vi "update_waypoints.vi"(11 "Mission in":refnum<class "Mission.lvclass">) -> (3 "Mission out":refnum<class "Mission.lvclass">)   [LabVIEW 2011, in "Mission.lvclass"]
uses:
  Mission.lvclass
  2 Globals/2 Global.vi
  Waypoint/Waypoint.lvclass
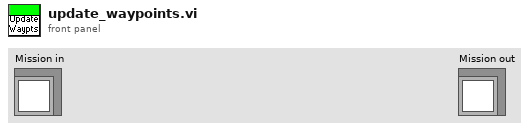
[diagram p1: front panel]
types:
  T1 = enum16{"Round Buoy", "Drive", "Pass Buoys", "Station Keeping"}
  T2 = typedef "UTM Location.ctl" = cluster{"UTM Zone":dbl, "Hemisphere":enum16{"North", "South"}, "East":dbl, "North":dbl}
  T3 = typedef "Waypoints List.ctl" = refnum<class "Waypoint.lvclass">[]
  T4 = typedef "Current Waypoint.ctl" = i32
  T5 = typedef "UTM Circle.ctl" = cluster{"UTM Zone":dbl, "Hemisphere":enum16{"North", "South"}, "East":dbl, "North":dbl, "Radius":dbl}
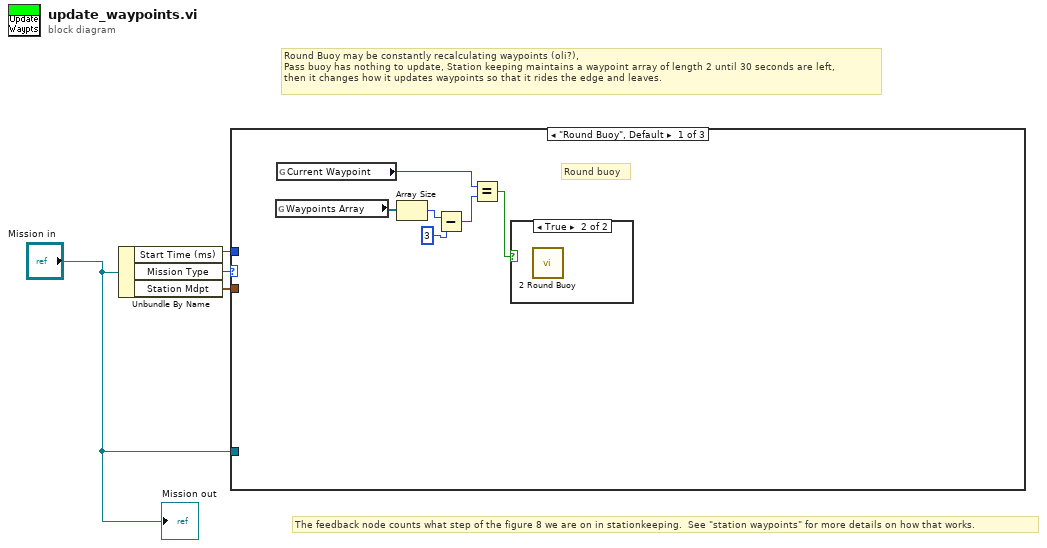
[diagram p0: block diagram]
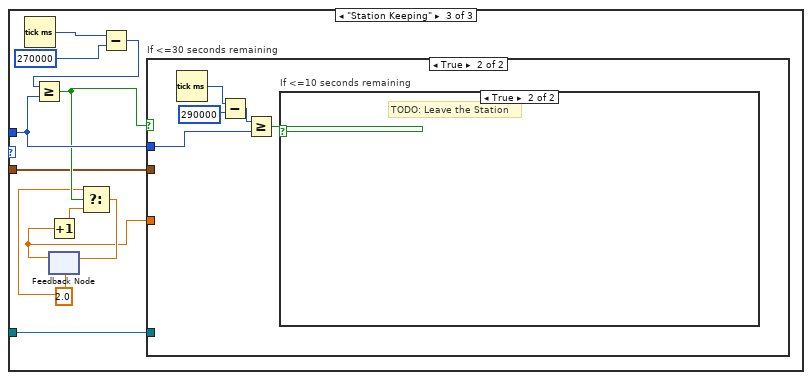
[diagram p4: hidden frame]
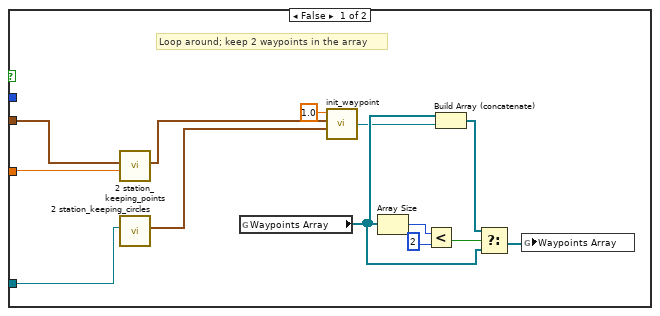
[diagram p5: hidden frame]
diagram:
  # "The feedback node counts what step of the figure 8 we are on in stationkeeping.  See \"station waypoints\" for more details on how that works."
  # "Round Buoy may be constantly recalculating waypoints (oli?),\nPass buoy has nothing to update, Station keeping maintains a waypoint array of length 2 until 30 seconds are left,\nthen it changes how it updates waypoints so that it rides the edge and leaves."
  n1 = Unbundle By Name("Mission in") -> ("Start Time (ms)"=w3:u32, "Mission Type"=w4:T1, "Station Mdpt"=w1:T2)
  n2 = case shown="\"Round Buoy\", Default" w4 {
    tunnel: w3 -> [_ _ w19]
    tunnel: "Mission in" -> [_ _ w12]
    tunnel: w1 -> [_ _ w11]
    frame "Round Buoy", Default {
      # "Round buoy"
      n3 = global read "2 Global.vi" "Waypoints Array"() -> (w9:T3)
      n4 = global read "2 Global.vi" "Current Waypoint"() -> (w7:T4)
      n5 = Array Size(array=w9) -> (size(s)=w8:i32)
      n6 = Subtract(x=w8, y=3) -> (x-y=w6:i32)
      n7 = Equal?(x=w7, y=w6) -> (x = y?=w5:bool)
      n8 = case shown="True" w5 {
        frame False {
        }
        frame True {
          n9 = call "2 Round Buoy.vi"() -> ()  [unwired: 12 in]
        }
      }
    }
    frame "Pass Buoys" {
    }
    frame "Station Keeping" {
      w15 = 2.0
      n10 = Tick Count (ms)() -> (millisecond timer value=w21:u32)
      n11 = feedback #1(w15) -> (w13:dbl)
      n12 = Increment(x=w13) -> (x+1=w16:dbl)
      n13 = Subtract(x=w21, y=u32 270000) -> (x-y=w18:u32)
      n14 = Greater Or Equal?(x=w18, y=w19) -> (x >= y?=w17:bool)
      n15 = Select(t=w15, s=w17, f=w16) -> (s? t:f=w14:dbl)
      n16 = feedback-in #1(w14) -> ()
      n17 = case "If <=30 seconds remaining" shown="True" w17 {
        tunnel: w19 -> [_ w36]
        tunnel: w13 -> [w29 _]
        tunnel: w12 -> [w25 _]
        tunnel: w11 -> [w24 _]
        frame False {
          # "Loop around; keep 2 waypoints in the array"
          n18 = call "2 station_keeping_points.vi"("Which Point?"=w29, "Midpoint"=w24) -> ("Waypoint"=w28:T2)  [unwired: 9 in]
          n19 = call "2 station_keeping_circles.vi"("Mission in"=w25) -> ("No Sail Circles"=w26:T5[])  [unwired: 10 in]
          n20 = global read "2 Global.vi" "Waypoints Array"() -> (w30:T3)
          n21 = call "init_waypoint.vi"("No Sail Circles"=w26, "Coords"=w28, "Tolerance (m)"=1.0 ("Tolerance (meters?)")) -> ("Waypoint Out"=w27:refnum<class "Waypoint.lvclass">)  [unwired: 8 in]
          n22 = Array Size(array=w30) -> (size(s)=w34:i32)
          n23 = Less?(x=w34, y=2) -> (x < y?=w32:bool)
          n24 = Build Array (concatenate)(w30, w27) -> (w31:T3)
          n25 = Select(t=w31, s=w32, f=w30) -> (s? t:f=w23:T3)
          n26 = global write "2 Global.vi" "Waypoints Array"(w23) -> ()
        }
        frame True {
          n27 = Tick Count (ms)() -> (millisecond timer value=w39:u32)
          n28 = Subtract(x=w39, y=u32 290000) -> (x-y=w37:u32)
          n29 = Greater Or Equal?(x=w37, y=w36) -> (x >= y?=w35:bool)
          n30 = case "If <=10 seconds remaining" shown="True" w35 {
            frame False {
              # "TODO: Ride a wall"
            }
            frame True {
              # "TODO: Leave the Station"
            }
          }
        }
      }
    }
  }
  "Mission out" <- "Mission in"
